vi "Counter 16 Bit iCmp (SubVI).vi"(1 "Max. Count":u16=65535, 2 "RESET":bool, 3 "Auto RESET":bool=TRUE, 11 "Enable":bool) -> (4 "Count":u16, 6 "Count Begin?":bool, 15 "Count End?":bool)   [LabVIEW 2015]
panel:
  # "Counter 16-Bit:\n\nCounts when Enable input is TRUE. Count value is 0-indexed."
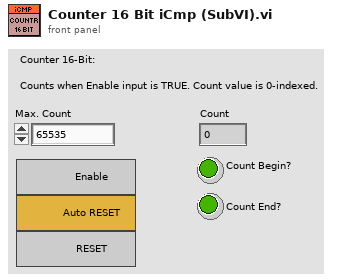
[diagram p1: front panel]
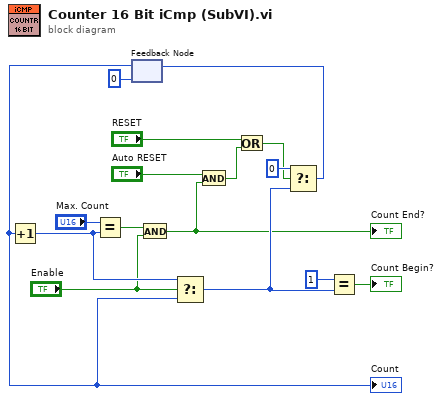
[diagram p0: block diagram]
diagram:
  n1 = feedback #1(u16 0) -> (w16:u16)
  "Count" <- w16
  n2 = Increment(x=w16) -> (x+1=w3:u16)
  n3 = Equal?(x="Max. Count", y=w3) -> (x = y?=w9:bool)
  n4 = And(x=w9, y="Enable") -> (x .and. y?=w2:bool)
  "Count End?" <- w2
  n5 = Select(t=w3, s="Enable", f=w16) -> (s? t:f=w7:u16)
  n6 = And(x="Auto RESET", y=w2) -> (x .and. y?=w5:bool)
  n7 = Or(x="RESET", y=w5) -> (x .or. y?=w4:bool)
  n8 = Select(t=u16 0, s=w4, f=w7) -> (s? t:f=w8:u16)
  n9 = feedback-in #1(w8) -> ()
  n10 = Equal?(x=u16 1, y=w7) -> (x = y?=→"Count Begin?":bool)
